vi "Do.vi"(8 "error in (no error)":errorcluster, 10 "Actor in":refnum<class "Actor.lvclass">, 11 "Pulse Acquired Result":refnum<class "Pulse Acquired Result.lvclass">) -> (0 "error out":errorcluster, 2 "Actor out":refnum<class "Actor.lvclass">)   [LabVIEW 2016, in "Pulse Acquired Result.lvclass"]
doc: "(<B>Filename</B>: Actor Framework.lvlib:Message.lvclass:Do.vi)\n\nDefines what a message does when it is received by an actor. Generally, a message instructs an actor to invoke one of its methods. By default, this method does nothing. A child class must override it to define behavior. Create a child class by using the Actor Framework Message Maker dialog box."
uses:
  Pulse Acquired Result.lvclass
  C:/github/Measure_core/Da Base Messages/Result Reply Msg/Result Reply Msg.lvclass
  <vilib>/ActorFramework/Actor/Actor.lvclass
  Application Controller/Application Controller.lvclass
  C:/Program Files/National Instruments/LabVIEW 2016/vi.lib/ActorFramework/Actor/Actor.lvclass
  Da Base Messages/Result Reply Msg/Result Reply Msg.lvclass/Result Reply Msg.ctl
  da Base Messages/Result Reply Msg/Read Result.vi
  Results/Acquired Result/Acquired Result.lvclass
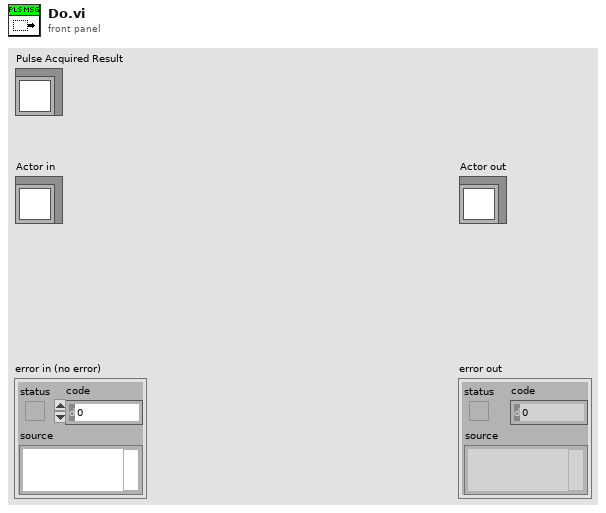
[diagram p1: front panel]
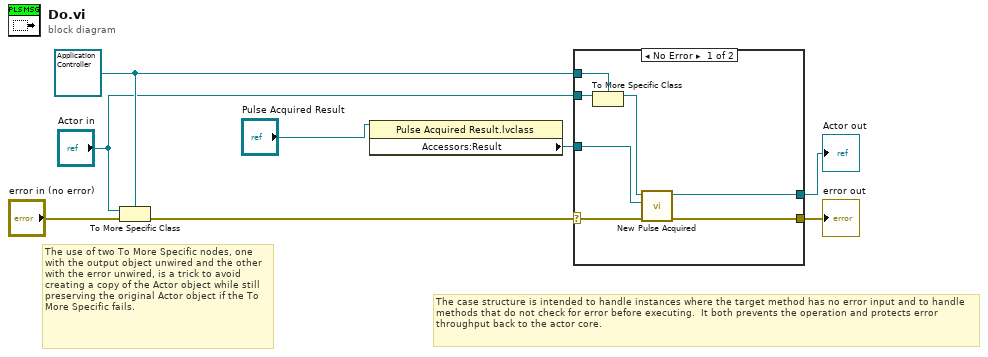
[diagram p0: block diagram]
diagram:
  w7 = refnum<class "Application Controller.lvclass"> refnum ("Actor in")
  # "The use of two To More Specific nodes, one with the output object unwired and the other with the error unwired, is a trick to avoid creating a copy of the Actor object while still preserving the original Actor object if the To More Specific fails."
  # "The case structure is intended to handle instances where the target method has no error input and to handle methods that do not check for error before executing.  It both prevents the operation and protects error throughput back to the actor core."
  n1 = To More Specific Class(target class=w7, reference="Actor in", error in="error in (no error)") -> (error out=w6:errorcluster)  [unwired: 1 out]
  n2 = property class="Pulse Acquired Result.lvclass"(reference="Pulse Acquired Result") -> ("Accessors:Result"=w8:refnum<class "Acquired Result.lvclass">)  [unwired: 1 in, 2 out]
  n3 = case shown="No Error" w6 {
    selector: w6 -> [w13 w17]
    tunnel: [w15 w17] -> w4
    tunnel: [w14 w16] -> w3
    tunnel: "Actor in" -> [w12 w16]
    tunnel: w7 -> [w11 _]
    tunnel: w8 -> [w9 _]
    frame No Error {
      n4 = To More Specific Class(target class=w11, reference=w12) -> (specific class reference=w10:refnum<class "Application Controller.lvclass">)  [unwired: 1 in, 1 out]
      n5 = call-dynamic "New Pulse Acquired.vi"("error in (no error)"=w13, "Acquired Result.lvclass"=w9, "Application Controller in"=w10) -> ("error out"=w15:errorcluster, "Application Controller out"=w14:refnum<class "Application Controller.lvclass">)  [unwired: 7 in]
    }
    frame Error {
      # "If type check fails, pass the original object out again."
    }
  }
  "error out" <- w4
  "Actor out" <- w3
